vi "triangle_wave_self_ex.vi"() -> ()   [LabVIEW 2017]
panel:
  out "Waveform Chart":dbl(graph)
  out "t":dbl
  out "T(s)":dbl
  in  "f(hz)":dbl
  in  "stop":bool
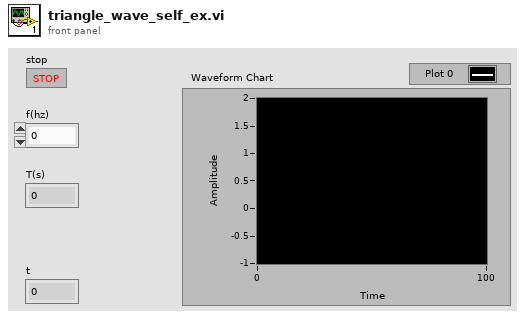
[diagram p1: front panel]
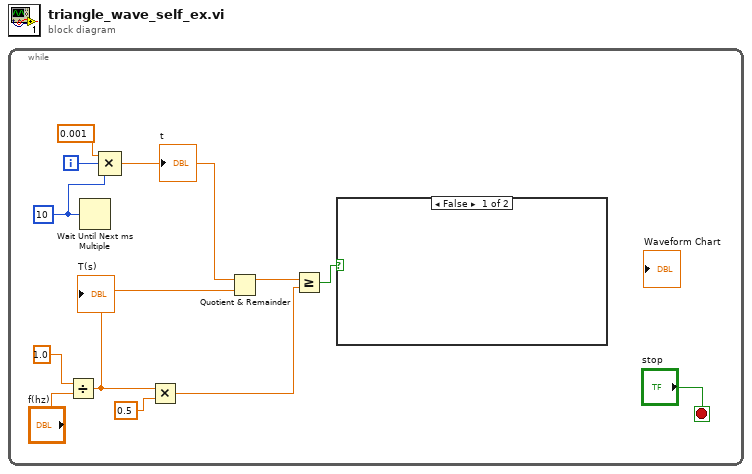
[diagram p0: block diagram]
diagram:
  n1 = while {
    i -> [w10]
    stop <- "stop" stop-if-true
    w11 = u32 10 ("millisecond multiple")
    n2 = Divide(x=1.0, y="f(hz)") -> (x/y=w5:dbl)
    "T(s)" <- w5
    n3 = Wait Until Next ms Multiple(millisecond multiple=w11) -> ()  [unwired: 1 out]
    n4 = Compound Arithmetic op=MULTIPLY(0.001, w10, w11) -> (w6:dbl)
    "t" <- w6
    n5 = Multiply(x=w5, y=0.5) -> (x*y=w2:dbl)
    n6 = Quotient & Remainder(x=w6, y=w5) -> (x-y*floor(x/y)=w3:dbl)  [unwired: 1 out]
    n7 = Greater Or Equal?(x=w3, y=w2) -> (x >= y?=w1:bool)
    n8 = case shown="False" w1 {
      frame False {
      }
      frame True {
      }
    }
  }
